vi "S2C_Shared_Proc_DefaultFP.vi"(8 "Error In":errorcluster, 11 "VI_Ref In":refnum<vi>) -> (0 "Error Out":errorcluster, 3 "VI_Ref Out":refnum<vi>)   [LabVIEW 2015]
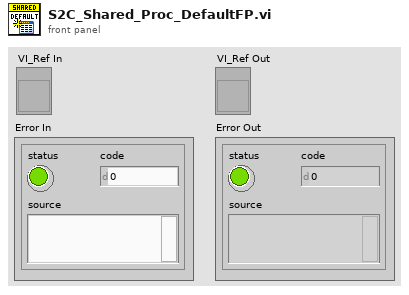
[diagram p1: front panel]
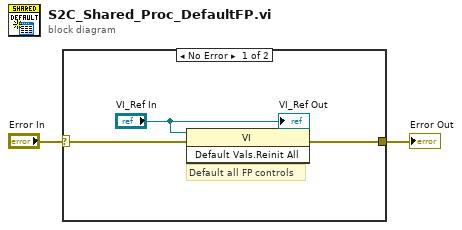
[diagram p0: block diagram]
diagram:
  n1 = case shown="No Error" "Error In" {
    selector: "Error In" -> [w5 w6]
    tunnel: [w3 w6] -> w1
    frame No Error {
      # "Default all FP controls"
      n2 = invoke class="VI" method="Default Vals.Reinit All"(reference="VI_Ref In", error in=w5) -> (error out=w3:errorcluster)  [unwired: 1 in, 2 out]
      "VI_Ref Out" <- "VI_Ref In"
    }
    frame Error {
    }
  }
  "Error Out" <- w1
